vi "Check Is Array.vi"(11 "Meta Data in":T1[](array[typedef])) -> (2 "Array":bool, 3 "Meta Data":T1[](array[typedef]))   [LabVIEW 2020, in "CDM-Config.lvlib" / "Config-Sqlite.lvclass"]
uses:
  Config-Sqlite.lvclass
  Config-Sqlite.lvclass/Config-Sqlite.ctl
  Meta Data.ctl
  CDM-Config.lvlib
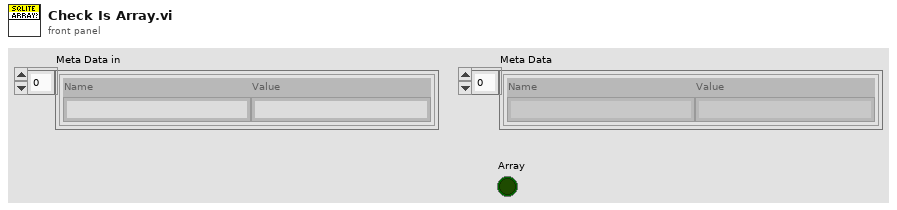
[diagram p1: front panel]
types:
  T1 = typedef "CDM-Config.lvlib/Meta Data.ctl" = cluster{"Name":string, "Value":string}
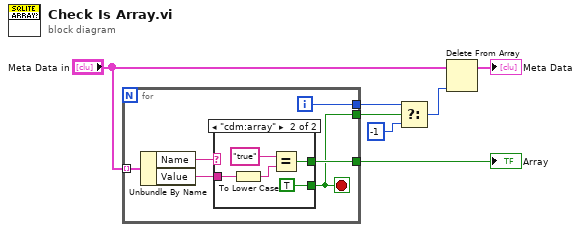
[diagram p0: block diagram]
diagram:
  n1 = for {
    tunnel: "Meta Data in" -> [w13] mode=indexing
    tunnel: [w9] -> w7
    tunnel: [w10] -> w6
    tunnel: [w8] -> w5
    i -> [w10]
    stop <- w8 stop-if-true
    n2 = Unbundle By Name(w13) -> ("Name"=w12:string, "Value"=w11:string)
    n3 = case shown="\"cdm:array\"" w12 {
      tunnel: w11 -> [_ w18]
      tunnel: [_ w15] -> w9
      tunnel: [_ TRUE] -> w8
      frame Default {
      }
      frame "cdm:array" {
        n4 = To Lower Case(string=w18) -> (all lower case string=w17:string)
        n5 = Equal?(x="true", y=w17) -> (x = y?=w15:bool)
      }
    }
  }
  "Array" <- w7
  n6 = Select(t=w6, s=w5, f=-1) -> (s? t:f=w1:i32)
  n7 = Delete From Array(array="Meta Data in", index=w1) -> (array with subset deleted=→"Meta Data":T1[])  [unwired: 1 in, 1 out]
